vi "LV2017CP.vi"() -> ()   [LabVIEW 2019]
doc: "This example performs a serial port write and a serial port read. The parameters set for the serial port must match the parameters of the connected instrument or device. The VISA Configure Serial Port VI sets the configuration parameters. The front panel displays the controls used to configure the basic parameters, such as baud rate, data bits, and parity. The VI passes the VISA resource name to other VIs that perform operations on that VISA resource. The VISA Write function sends a command to the serial device and the VISA Read function returns data based on the command. The VISA Close function then closes the reference to the serial device. It is important to close the reference; otherwise, further communication through that port might not be possible."
uses:
  <vilib>/Instr/_visa.llb/VISA Configure Serial Port (Instr).vi
  Serial - Settings.ctl
panel:
  in  "[exception action] (none:0)":i32(ring) items=["no exception", "cancel error on match", "set error on match"]
  out "read buffer 6":string
  out "read buffer 5":string
  out "read buffer 4":string
  out "read buffer 3":string
  out "read buffer 2":string
  out "read buffer":string
  in  "write buffer 2":string="\u0002\u0003RÑ\u0000\u0002„¹"
  in  "write buffer":string="\u0002\u0010Uï\u0000\u0002\u0004\u0000\u0000 @\b@"
  out "Answer to Write Command":string
  out "Floating Point 3":sgl
  out "Speed Ref in 21200":string
  out "Floating Point 2":sgl
  out "Speed Ref in Monitor":string
  out "I_d":sgl(graph)
  out "I_q":sgl(graph)
  out "Power(kW)":sgl(graph)
  out "Current(I)":sgl(graph)
  in  "file path (dialog if empty)":path=path "C:/Users/arda/Documents/GitHub/labviewtestbench/100 second data point.txt"
  in  "nominal rpm of the motor":sgl=750.0
  in  "Tyre Diameter(m)":sgl=0.5
  out "Real RPM":sgl(graph)=-0.028610228
  in  "Enum":T1(ring)
  in  "Continuous Connection(Def:ON)":bool
  out "Real Torque":sgl(graph)=-0.8946457
  in  "Finish session(Def:Off/False)":bool=TRUE
  in  "Connectivity Check (Def:Off)":bool
  in  "timeout (10sec)":u32=10000
  out "connection check":u8[](array[numeric])=[0, 0, 0, 2]
  in  "Enable Termination\nChar (T)":bool
  in  "connection_verification":string="\u0002\u0003Fm\u0000\u0002@­"
  out "Serial Settings:Wire Mode":i8(ring)=-128 items=["Unknown"=-1, "RS485/Wire4"=0, "RS485/Wire2-EchoDTR"=1, "RS485/Wire2-CtrlDTR"=2, "RS485/Wire2-Auto"=3, "RS232/DTE"=-128, "RS232/DCE"=-127, "RS232/Auto"=-126]
  out "message":string="No Error"
  in  "Serial Settings":T2={"baud rate"=19200, "data bits"=8, "parity"=enum."Even", "stop bits"=10, "flow control"=0} {"flow control" items=["None"=0, "XON/XOFF"=1, "RTS/CTS"=2, "DTR/DSR"=4]; "stop bits" items=["1.0"=10, "1.5"=15, "2.0"=20]; "data bits" min=5 max=8 step=1; "baud rate" items=["75"=75, "110"=110, "134"=134, "150"=150, "300"=300, "600"=600, "1200"=1200, "1800"=1800, "2400"=2400, "4800"=4800, "7200"=7200, "19600"=9600, "14400"=14400, "19200"=19200, "28800"=28800, "38400"=38400, "56000"=56000, "57600"=57600, "115200"=115200, "128000"=128000, "230400"=230400]}
  in  "VISA resource name":refnum<visa-resource-name>="COM8"
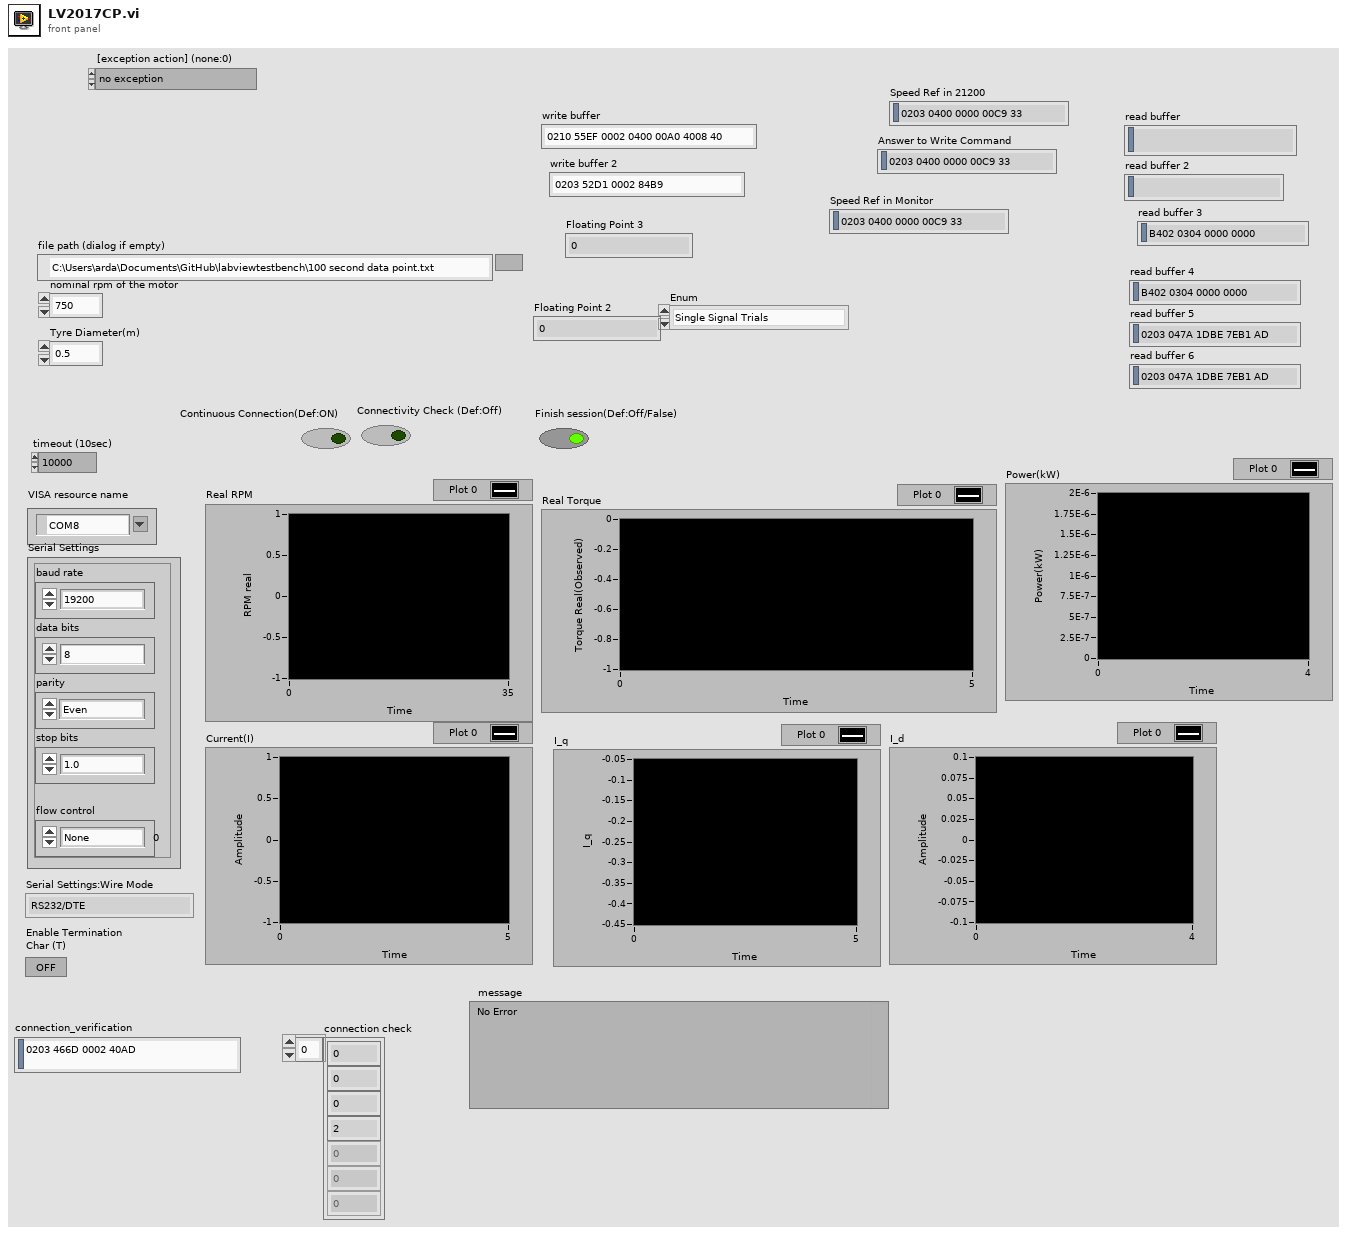
[diagram p1: front panel]
types:
  T1 = enum16{"Single Signal Trials", "Default", "Alarm Reset", "Write Save Command", "Drive Reset"}
  T2 = typedef "Serial - Settings.ctl" = cluster{"baud rate":u32, "data bits":u16, "parity":enum16{"None", "Odd", "Even", "Mark", "Space"}, "stop bits":u16, "flow control":u16}
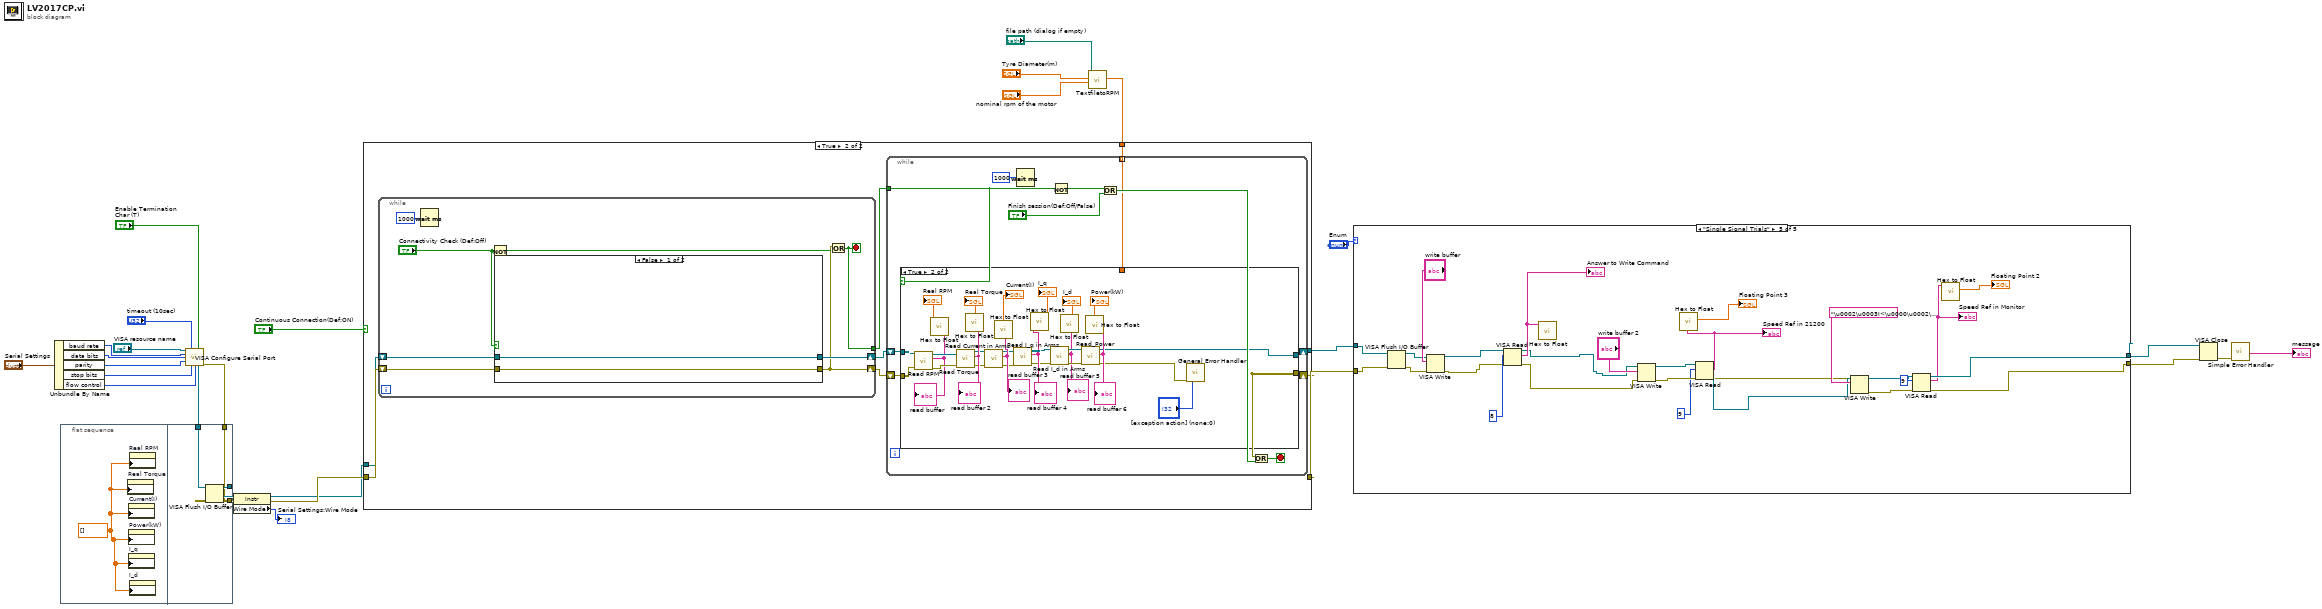
[diagram p0: block diagram]
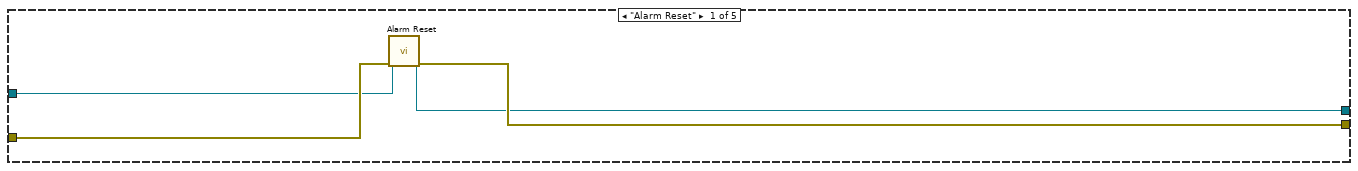
[diagram p2: hidden frame]
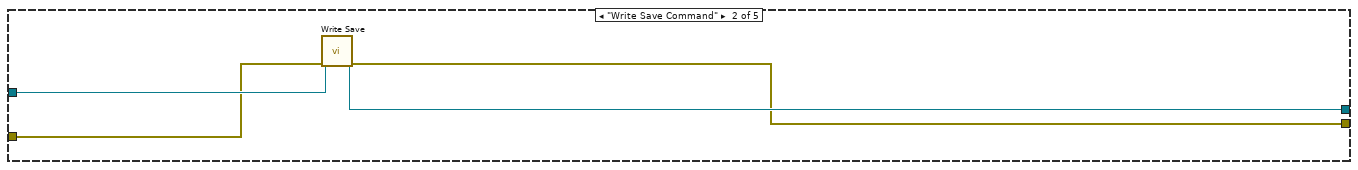
[diagram p3: hidden frame]
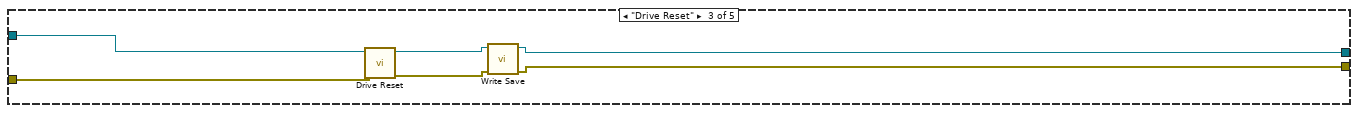
[diagram p4: hidden frame]
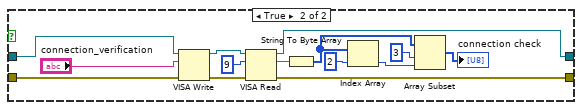
[diagram p7: hidden frame]
diagram:
  n1 = Unbundle By Name("Serial Settings") -> ("baud rate"=w22:u32, "data bits"=w26:u16, "parity"=w25:enum16{"None", "Odd", "Even", "Mark", "Space"}, "stop bits"=w24:u16, "flow control"=w23:u16)
  n2 = flat-sequence {
    tunnel: [w33] -> w19
    tunnel: [w32] -> w18
    tunnel: w17 -> [w31]
    tunnel: w16 -> [w30]
    frame #0 {
      w29 = sgl[] [] ("History Data")
      n3 = property on="Real Torque" class="WFChart (strict)"("History Data"=w29) -> ()  [unwired: 2 in, 2 out]
      n4 = property on="Current(I)" class="WFChart (strict)"("History Data"=w29) -> ()  [unwired: 2 in, 2 out]
      n5 = property on="Power(kW)" class="WFChart (strict)"("History Data"=w29) -> ()  [unwired: 2 in, 2 out]
      n6 = property on="I_q" class="WFChart (strict)"("History Data"=w29) -> ()  [unwired: 2 in, 2 out]
      n7 = property on="Real RPM" class="WFChart (strict)"("History Data"=w29) -> ()  [unwired: 2 in, 2 out]
      n8 = property on="I_d" class="WFChart (strict)"("History Data"=w29) -> ()  [unwired: 2 in, 2 out]
    }
    frame #1 {
      n9 = VISA Flush I/O Buffer(VISA resource name=w31, error in (no error)=w30) -> (VISA resource name out=w32:refnum<visa-resource-name>, error out=w33:errorcluster)  [unwired: 1 in]
    }
  }
  n10 = call-poly "VISA Configure Serial Port"("VISA resource name"="VISA resource name", "timeout (10sec)"="timeout (10sec)", "Enable Termination\nChar (T)"="Enable Termination\nChar (T)", "baud rate (9600)"=w22, "data bits (8)"=w26, "parity (0:none)"=w25, "stop bits (10: 1 bit)"=w24, "flow control (0:none)"=w23) -> ("VISA resource name out"=w17:refnum<visa-resource-name>, "error out"=w16:errorcluster)  [unwired: 1 in, 5 out]
  n11 = property class="Instr"(reference=w18, error in=w19) -> (reference out=w13:refnum<visa-resource-name>, error out=w14:errorcluster, "Wire Mode"=→"Serial Settings:Wire Mode":i16)
  n12 = call "TextfiletoRPM.vi"("nominal rpm of the motor"="nominal rpm of the motor", "Tyre Diameter(m)"="Tyre Diameter(m)", "file path (dialog if empty)"="file path (dialog if empty)") -> ("Array"=w4:dbl[])  [unwired: 7 in, 1 out]
  n13 = case shown="True" "Continuous Connection(Def:ON)" {
    tunnel: w14 -> [w34 w43]
    tunnel: w13 -> [w35 w42]
    tunnel: [w35 w39] -> w9
    tunnel: [w34 w38] -> w10
    tunnel: w4 -> [_ w36]
    frame False {
    }
    frame True {
      n14 = while {
        shift-right: [w51] -> w41
        shift-left: w42 -> [w50]
        shift-right: [w48] -> w40
        shift-left: w43 -> [w49]
        tunnel: [w44] -> w37
        stop <- w44 stop-if-true
        n15 = Wait (ms)(milliseconds to wait=u32 1000) -> ()  [unwired: 1 out]
        n16 = Not(x="Connectivity Check (Def:Off)") -> (.not. x?=w45:bool)
        n17 = case shown="False" "Connectivity Check (Def:Off)" {
          tunnel: [w53 w67] -> w51
          tunnel: w50 -> [w53 w66]
          tunnel: w49 -> [w52 w65]
          tunnel: [w52 w64] -> w48
          frame False {
          }
          frame True {
            n18 = VISA Write(VISA resource name=w66, write buffer="connection_verification", error in (no error)=w65) -> (VISA resource name out=w63:refnum<visa-resource-name>, error out=w61:errorcluster)  [unwired: 1 out]
            n19 = VISA Read(VISA resource name=w63, byte count=u32 9, error in (no error)=w61) -> (VISA resource name out=w67:refnum<visa-resource-name>, read buffer=w55:string, error out=w64:errorcluster)  [unwired: 1 out]
            n20 = String To Byte Array(string=w55) -> (unsigned byte array=w59:u8[])
            n21 = Index Array(array=w59, index=2) -> (element=w56:u8)
            n22 = Array Subset(array=w59, index=3 ("length"), length=w56) -> (→"connection check":u8[])
          }
        }
        n23 = Or(x=w48, y=w45) -> (x .or. y?=w44:bool)
      }
      n24 = while {
        shift-right: [w76] -> w39
        shift-left: w41 -> [w78]
        shift-right: [w74] -> w38
        shift-left: w40 -> [w77]
        tunnel: w37 -> [w73]
        tunnel: w36 -> [w68] mode=indexing
        stop <- w70 stop-if-true
        n25 = case shown="True" w73 {
          tunnel: w78 -> [w80 w102]
          tunnel: w77 -> [w79 w101]
          tunnel: [w80 w83] -> w76
          tunnel: [w79 _] -> w74
          tunnel: w68 -> [_ _]
          frame False {
          }
          frame True {
            n26 = call "Read RPM.vi"("error in (no error)"=w101, "VISA resource name"=w102) -> ("error out"=w103:errorcluster, "read buffer"=w100:string, "VISA resource name out"=w104:refnum<visa-resource-name>)  [unwired: 7 in]
            "read buffer" <- w100
            n27 = call "Hex to Float.vi"("read buffer in"=w100) -> ("Floating Point"=→"Real RPM":sgl)  [unwired: 9 in, 1 out]
            n28 = call "Read Torque.vi"("error in (no error)"=w103, "VISA Refnum in"=w104) -> ("error out"=w95:errorcluster, "read buffer"=w107:string, "VISA Refnum out"=w96:refnum<visa-resource-name>)  [unwired: 7 in]
            "read buffer 2" <- w107
            n29 = call "Hex to Float.vi"("read buffer in"=w107) -> ("Floating Point"=→"Real Torque":sgl)  [unwired: 9 in, 1 out]
            n30 = call "Read Current in Arms.vi"("error in (no error)"=w95, "VISA Refnum in"=w96) -> ("error out"=w92:errorcluster, "read buffer"=w94:string, "VISA Refnum out"=w93:refnum<visa-resource-name>)  [unwired: 7 in]
            "read buffer 3" <- w94
            n31 = call "Hex to Float.vi"("read buffer in"=w94) -> ("Floating Point"=→"Current(I)":sgl)  [unwired: 9 in, 1 out]
            n32 = call "Read I_q in Arms.vi"("error in (no error)"=w92, "VISA Refnum in"=w93) -> ("error out"=w88:errorcluster, "read buffer"=w91:string, "VISA Refnum out"=w89:refnum<visa-resource-name>)  [unwired: 7 in]
            "read buffer 4" <- w91
            n33 = call "Hex to Float.vi"("read buffer in"=w91) -> ("Floating Point"=→"I_q":sgl)  [unwired: 9 in, 1 out]
            n34 = call "Read I_d in Arms.vi"("error in (no error)"=w88, "VISA Refnum in"=w89) -> ("error out"=w86:errorcluster, "read buffer"=w85:string, "VISA Refnum out"=w87:refnum<visa-resource-name>)  [unwired: 7 in]
            "read buffer 5" <- w85
            n35 = call "Hex to Float.vi"("read buffer in"=w85) -> ("Floating Point"=→"I_d":sgl)  [unwired: 9 in, 1 out]
            n36 = call "Read_Power.vi"("error in (no error)"=w86, "VISA Refnum in"=w87) -> ("error out"=w82:errorcluster, "read buffer"=w98:string, "VISA Refnum out"=w83:refnum<visa-resource-name>)  [unwired: 7 in]
            "read buffer 6" <- w98
            n37 = call "Hex to Float.vi"("read buffer in"=w98) -> ("Floating Point"=→"Power(kW)":sgl)  [unwired: 9 in, 1 out]
            n38 = call <vilib>:"General Error Handler.vi"("error in (no error)"=w82, "[exception action] (none:0)"="[exception action] (none:0)") -> ()  [unwired: 9 in, 5 out]
          }
        }
        n39 = Wait (ms)(milliseconds to wait=u32 1000) -> ()  [unwired: 1 out]
        n40 = Not(x=w73) -> (.not. x?=w72:bool)
        n41 = Or(x=w72, y="Finish session(Def:Off/False)") -> (x .or. y?=w69:bool)
        n42 = Or(x=w74, y=w69) -> (x .or. y?=w70:bool)
      }
    }
  }
  n43 = case shown="\"Single Signal Trials\"" "Enum" {
    tunnel: w10 -> [w111 w114 w120 w122 w126]
    tunnel: w9 -> [w110 w115 w121 w123 w127]
    tunnel: [w109 w112 w116 w122 w149] -> w8
    tunnel: [w108 w113 w117 w123 w150] -> w7
    frame "Alarm Reset" {
      n44 = call "Alarm Reset.vi"("error in (no error)"=w111, "VISA Refnum in"=w110) -> ("error out"=w109:errorcluster, "VISA Refnum out"=w108:refnum<visa-resource-name>)  [unwired: 7 in, 1 out]
    }
    frame "Write Save Command" {
      n45 = call "Write Save.vi"("error in (no error)"=w114, "VISA Refnum in"=w115) -> ("error out"=w112:errorcluster, "VISA Refnum out"=w113:refnum<visa-resource-name>)  [unwired: 7 in, 1 out]
    }
    frame "Drive Reset" {
      n46 = call "Drive Reset.vi"("error in (no error)"=w120, "VISA Refnum in"=w121) -> ("error out"=w118:errorcluster, "VISA Refnum out"=w119:refnum<visa-resource-name>)  [unwired: 7 in, 1 out]
      n47 = call "Write Save.vi"("error in (no error)"=w118, "VISA Refnum in"=w119) -> ("error out"=w116:errorcluster, "VISA Refnum out"=w117:refnum<visa-resource-name>)  [unwired: 7 in, 1 out]
    }
    frame "Default" {
    }
    frame "Single Signal Trials" {
      n48 = VISA Flush I/O Buffer(VISA resource name=w127, error in (no error)=w126) -> (VISA resource name out=w124:refnum<visa-resource-name>, error out=w125:errorcluster)  [unwired: 1 in]
      n49 = VISA Write(VISA resource name=w124, write buffer="write buffer", error in (no error)=w125) -> (VISA resource name out=w129:refnum<visa-resource-name>, error out=w128:errorcluster)  [unwired: 1 out]
      n50 = VISA Read(VISA resource name=w129, byte count=u32 8, error in (no error)=w128) -> (VISA resource name out=w131:refnum<visa-resource-name>, read buffer=w132:string, error out=w130:errorcluster)  [unwired: 1 out]
      "Answer to Write Command" <- w132
      n51 = call "Hex to Float.vi"("read buffer in"=w132) -> ()  [unwired: 9 in, 2 out]
      n52 = VISA Write(VISA resource name=w131, write buffer="write buffer 2", error in (no error)=w130) -> (VISA resource name out=w139:refnum<visa-resource-name>, error out=w140:errorcluster)  [unwired: 1 out]
      n53 = VISA Read(VISA resource name=w139, byte count=u32 9, error in (no error)=w140) -> (VISA resource name out=w135:refnum<visa-resource-name>, read buffer=w137:string, error out=w134:errorcluster)  [unwired: 1 out]
      "Speed Ref in 21200" <- w137
      n54 = call "Hex to Float.vi"("read buffer in"=w137) -> ("Floating Point"=→"Floating Point 3":sgl)  [unwired: 9 in, 1 out]
      n55 = VISA Write(VISA resource name=w135, write buffer="\u0002\u0003I<\u0000\u0002\u0012h", error in (no error)=w134) -> (VISA resource name out=w146:refnum<visa-resource-name>, error out=w147:errorcluster)  [unwired: 1 out]
      n56 = VISA Read(VISA resource name=w146, byte count=u32 9, error in (no error)=w147) -> (VISA resource name out=w150:refnum<visa-resource-name>, read buffer=w144:string, error out=w149:errorcluster)  [unwired: 1 out]
      "Speed Ref in Monitor" <- w144
      n57 = call "Hex to Float.vi"("read buffer in"=w144) -> ("Floating Point"=→"Floating Point 2":sgl)  [unwired: 9 in, 1 out]
    }
  }
  n58 = VISA Close(VISA resource name=w7, error in (no error)=w8) -> (error out=w12:errorcluster)
  n59 = call <vilib>:"Simple Error Handler.vi"("error in (no error)"=w12) -> ("message"=→"message":string)  [unwired: 1 in, 7 out]
